vi "Rename First File.vi"(11 "output cluster":T1) -> ()   [LabVIEW 2024]
panel:
  out "concatenated string 2":string
  out "concatenated string":string
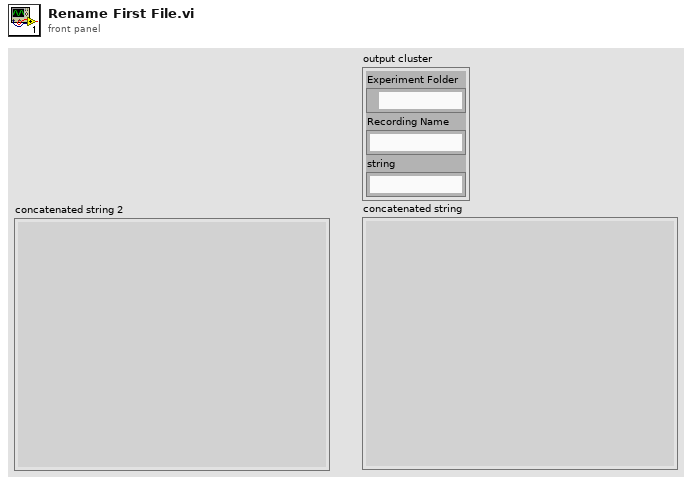
[diagram p1: front panel]
types:
  T1 = cluster{"Experiment Folder":path, "Recording Name":string, "string":string}
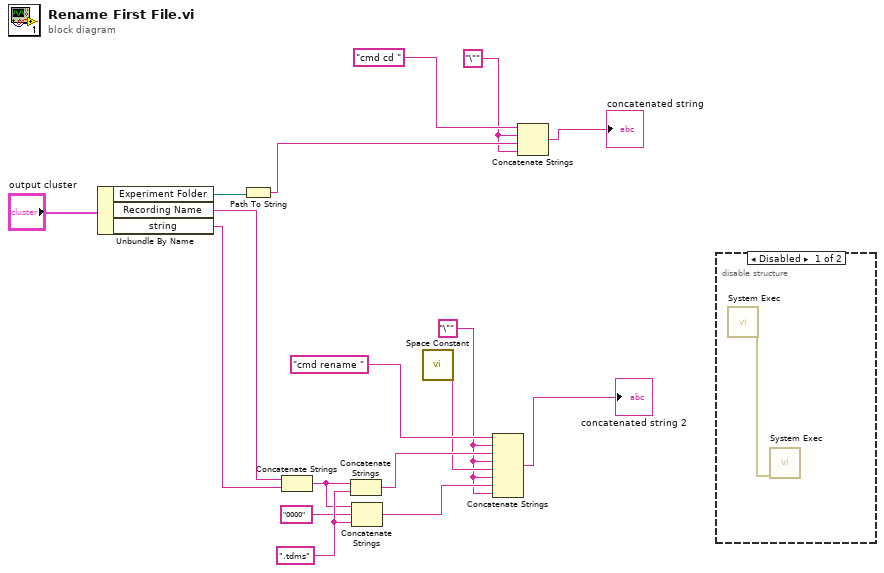
[diagram p0: block diagram]
diagram:
  w11 = ".tdms" ("string")
  w6 = "\""
  w13 = "\""
  n1 = Unbundle By Name("output cluster") -> ("Experiment Folder"=w16:path, "Recording Name"=w2:string, "string"=w1:string)
  n2 = Path To String(path=w16) -> (string=w14:string)
  n3 = Concatenate Strings(w2, w1) -> (w5:string)
  n4 = Concatenate Strings(w5, w11) -> (w9:string)
  n5 = Concatenate Strings(w5, "0000" ("string"), w11) -> (w7:string)
  n6 = call <vilib>:"Space Constant.vi"() -> ("String"=w8:string)
  n7 = Concatenate Strings("cmd rename ", w6, w9, w6, w8, w6, w7, w6) -> (→"concatenated string 2":string)
  n8 = Concatenate Strings("cmd cd ", w13, w14, w13) -> (→"concatenated string":string)
  n9 = disable-structure shown="Disabled" {
    frame Disabled {
      n10 = call <vilib>:"System Exec.vi"() -> ("error out"=w18:errorcluster)  [unwired: 8 in, 3 out]
      n11 = call <vilib>:"System Exec.vi"("error in (no error)"=w18) -> ()  [unwired: 7 in, 4 out]
    }
    frame Enabled {
    }
  }
